vi "Apply High Speed Capture.vi"(8 "error in":errorcluster, 11 "3300 in":refnum<class "3300.lvclass">) -> (0 "error out":errorcluster, 3 "3300 out":refnum<class "3300.lvclass">)   [LabVIEW 2019, in "3300.lvlib" / "3300.lvclass"]
doc: "Apply default timing and windowing settings. This configures each Eload module to Hanning window 10 samples within a 10us sample interval on measurement queries with triggering disabled."
uses:
  Library/3300.lvclass
  C:/Users/Public/Documents/Development/builds/Instruments/Electronic Load.lvlibp/Library/Electronic Load.lvclass
  builds/Instruments/Electronic Load.lvlibp/Accessors/Read Available Channels.vi
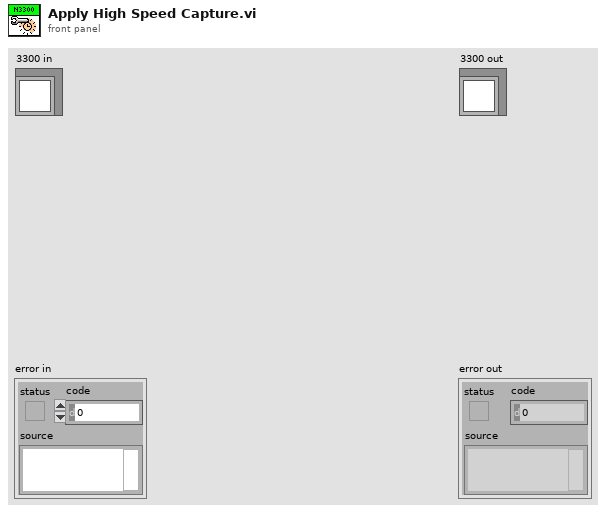
[diagram p1: front panel]
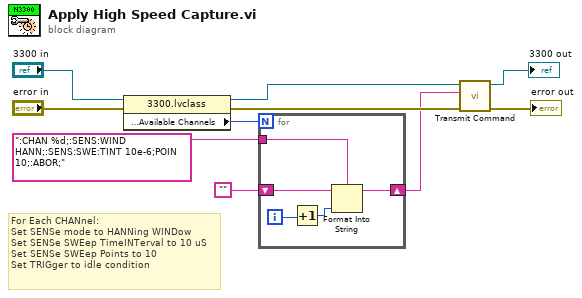
[diagram p0: block diagram]
diagram:
  # "For Each CHANnel:\nSet SENSe mode to HANNing WINDow\nSet SENSe SWEep TimeINTerval to 10 uS\nSet SENSe SWEep Points to 10\nSet TRIGger to idle condition"
  n1 = property class="3300.lvclass"(reference="3300 in", error in="error in") -> (reference out=w6:refnum<class "3300.lvclass">, error out=w4:errorcluster, "Accessors:Configuration:Available Channels"=w1:i32)
  n2 = for {
    N: w1 -> [_]
    tunnel: ":CHAN %d;:SENS:WIND HANN;:SENS:SWE:TINT 10e-6;POIN 10;:ABOR;" -> [w14]
    shift-right: [w11] -> w2
    shift-left: "" -> [w15]
    i -> [w13]
    n3 = Increment(x=w13) -> (x+1=w12:i32)
    n4 = Format Into String(format string=w14, initial string=w15, w12) -> (resulting string=w11:string)  [unwired: 1 in, 1 out]
  }
  n5 = call "Transmit Command.vi"("error in"=w4, "Command"=w2, "3300 in"=w6) -> ("error out"=→"error out":errorcluster, "3300 out"=→"3300 out":refnum<class "3300.lvclass">)  [unwired: 7 in]
